vi "Select U8 values.vi"(10 "Unput U8":u8) -> (2 "output I32":i32)   [LabVIEW 2015, in "DDC_7976R_v1.lvlib"]
uses:
  DDC_7976R_v1.lvlib
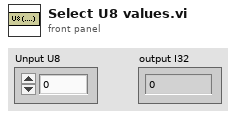
[diagram p1: front panel]
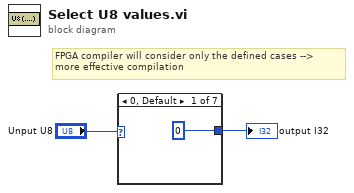
[diagram p0: block diagram]
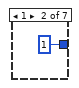
[diagram p2: hidden frame]
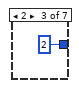
[diagram p3: hidden frame]
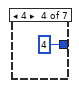
[diagram p4: hidden frame]
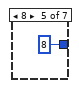
[diagram p5: hidden frame]
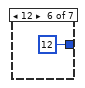
[diagram p6: hidden frame]
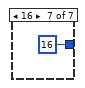
[diagram p7: hidden frame]
diagram:
  # "FPGA compiler will consider only the defined cases -->\nmore effective compilation"
  n1 = case shown="0, Default" "Unput U8" {
    tunnel: [0 1 2 4 8 12 16] -> w2
    frame 0, Default {
    }
    frame 1 {
    }
    frame 2 {
    }
    frame 4 {
    }
    frame 8 {
    }
    frame 12 {
    }
    frame 16 {
    }
  }
  "output I32" <- w2
